vi "libssh2_session_handshake_socket - invalid session - no error 1097.vi"() -> ()   [LabVIEW 2013, in "libssh2_tests.lvlib"]
uses:
  libssh2_tests.lvlib
  libssh2/Session Refnum.ctl
  libssh2/libssh2_init_default.vi
  <vilib>/Utility/error.llb/General Error Handler.vi
  <vilib>/addons/_JKI Toolkits/Caraya/classes/Assert/Assert.vi
  <vilib>/addons/_JKI Toolkits/Caraya/classes/Assert/Assert Not Error.vi
  <vilib>/addons/_JKI Toolkits/Caraya/classes/Test/Test.lvclass
  libssh2/libssh2.lvlib
panel:
  out "error out":errorcluster
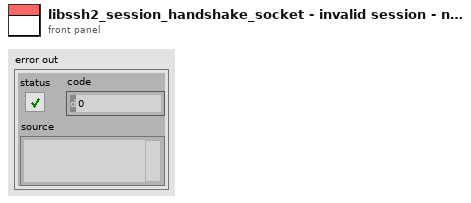
[diagram p1: front panel]
types:
  T1 = typedef "libssh2.lvlib/Session Refnum.ctl" = refnum<k1>
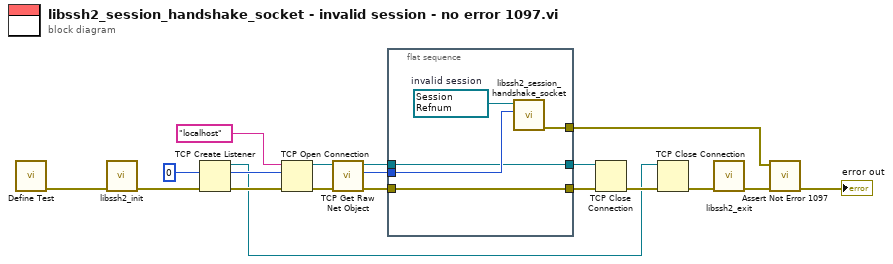
[diagram p0: block diagram]
diagram:
  n1 = call <vilib>:"Define Test.vi"() -> ("error out"=w18:errorcluster)  [unwired: 10 in, 1 out]
  n2 = call-poly "libssh2_init.vi"("error in (no error)"=w18) -> ("error out"=w15:errorcluster)  [unwired: 10 in]
  n3 = TCP Create Listener(8:w15, 10:u16 0 ("remote port or service name")) -> (0:w14:errorcluster, 2:w7:u16, 3:w2:refnum<k5>)  [unwired: 3 in]
  n4 = TCP Open Connection(address="localhost", remote port or service name=w7, error in (no error)=w14) -> (connection ID=w10:refnum<k5>, error out=w12:errorcluster)  [unwired: 2 in]
  n5 = call <vilib>:"TCP Get Raw Net Object.vi"("error in (no error)"=w12, "connection ID"=w10) -> ("error out"=w11:errorcluster, "raw net object"=w9:u64, "connection ID out"=w6:refnum<k5>)  [unwired: 7 in]
  n6 = flat-sequence {
    tunnel: [w23] -> w16
    tunnel: w11 -> [w23]
    tunnel: [w22] -> w1
    tunnel: w9 -> [w21]
    tunnel: w6 -> [w20]
    tunnel: [w20] -> w5
    frame #0 {
      w24 = T1 refnum items=["Session"]  # invalid session
      n7 = call "libssh2_session_handshake_socket.vi"("socket"=w21, "session"=w24) -> ("error out"=w22:errorcluster)  [unwired: 9 in]
    }
  }
  n8 = TCP Close Connection(connection ID=w5, error in (no error)=w16) -> (error out=w4:errorcluster)  [unwired: 1 in, 1 out]
  n9 = TCP Close Connection(connection ID=w2, error in (no error)=w4) -> (error out=w3:errorcluster)  [unwired: 1 in, 1 out]
  n10 = call "libssh2_exit.vi"("error in (no error)"=w3) -> ("error out"=w17:errorcluster)  [unwired: 10 in]
  n11 = call "Assert Not Error 1097.vi"("error in (no error)"=w17, "actual value"=w1) -> ("error out"=→"error out":errorcluster)  [unwired: 9 in]
